vi "Configuration Keys.vi"(8 "error in":errorcluster, 11 "Multimeter in":refnum<class "Multimeter.lvclass">) -> (0 "error out":errorcluster, 2 "Required Keys":string[](array[string]), 3 "Multimeter out":refnum<class "Multimeter.lvclass">)   [LabVIEW 2019, in "Multimeter.lvlib" / "Multimeter.lvclass"]
doc: "Configuration Keys is a dynamic dispatch VI that reads a full inheritance chain's required key list.\n\nThis means each instrument must override this vi, and call the parent method . The end result is a comprehensive list of required keys that must be present in an instrument's config.ini file to correctly function."
uses:
  Library/Multimeter.lvclass
  builds/Instruments/Instruments.lvlibp/Library/Instruments.lvclass
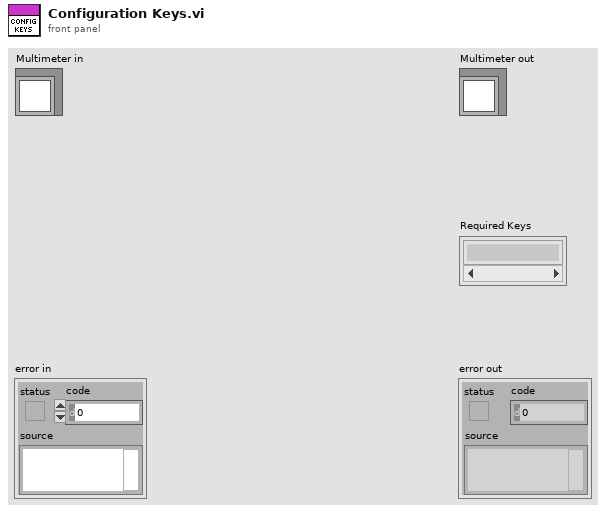
[diagram p1: front panel]
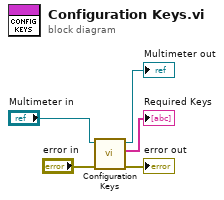
[diagram p0: block diagram]
diagram:
  n1 = call-parent "Configuration Keys.vi"("error in"="error in", "Instruments in"="Multimeter in") -> ("error out"=→"error out":errorcluster, "Required Keys"=→"Required Keys":string[], "Instruments out"=→"Multimeter out":refnum<class "Multimeter.lvclass">)  [unwired: 7 in]
